vi "Main.vi"() -> ()   [LabVIEW 2018, in "HW Interaction.lvlib"]
doc: "This template is based off of the Queued Message Handler design pattern and the Queued Message Handler project template that ships with LabVIEW.\n\nThe main difference is that the queue is private to this module and communication between modules is performed via Broadcast and Request events.\n\nRequest events are wrapped in public API methods and are handled in the Event Handling Loop (EHL) of this VI. Any module can register for Broadcast events sent by this module. The EHL generates messages based on user interface actions.\n\nThe Message Handling Loop (MHL) processes messages generated by the EHL, or by other messages. The messages are string values, so new messages can be added easily to the Message Cases case structure in the MHL. Each message cluster can also provide an optional value for Message Data, which is a variant that can be converted to whatever message-specific data is required.\n_____\nBased on Delacor QMH Project Template 4.2.1.64."
uses:
  HW Interaction.lvlib
  <vilib>/Delacor/Delacor QMH/Libraries/Module Admin_class/Delacor_lib_QMH_Module Admin.lvclass
  Private API/Data.lvclass
  <vilib>/Delacor/Delacor QMH/Libraries/Message Queue_class/Delacor_lib_QMH_Message Queue.lvclass/Delacor_lib_QMH_Message Queue.ctl
  Stop Argument--cluster.ctl
  <vilib>/Delacor/Delacor QMH/Libraries/Module Admin_class/Delacor_lib_QMH_Module Admin.lvclass/Delacor_lib_QMH_Module Admin.ctl
  Prepare to Exit Argument--cluster.ctl
  HW Init Argument--cluster.ctl
  Public API/Typedefs/CTL_Port_connection_type.ctl
  SubVi's/Controls/CTL_Acquisition_speed_selector.ctl
  <vilib>/Utility/miscctls.llb/LVPointTypeDef.ctl
  Private API/Data.lvclass/Data.ctl
  HW Init Outcome Argument--cluster.ctl
  Public API/Typedefs/CTL_Sensor_board_type_(size).ctl
  Private API/Typedefs/CTL_HW_Interaction_Commands.ctl
  <vilib>/Delacor/Delacor QMH/Libraries/Message Queue_class/Delacor_lib_QMH_Enqueue Message (Single).vi
  <vilib>/Delacor/Delacor QMH/Libraries/Module Admin_class/Delacor_lib_QMH_Get External Launch.vi
  Private API/Methods/Write Status.vi
  Private API/Methods/Write FW Version.vi
  Private API/Methods/Write Sync capability.vi
  Private API/Methods/Write Port Opened.vi
  Private API/Methods/Write Sensor board type.vi
  Private API/Methods/Write HW set FPS.vi
  Private API/Methods/Write Serial Port.vi
  Private API/Methods/Read All Port Info.vi
  <vilib>/Utility/error.llb/Error Cluster From Error Code.vi
  <vilib>/ErrorRing/Error Ring.xnode
  <vilib>/Delacor/Delacor QMH/Libraries/Message Queue_class/Delacor_lib_QMH_Message Queue.lvclass
  Common_Resources.lvlib
panel:
  in  "Simulate MHL Error":bool
  in  "Simulate EHL Error":bool
  out "error out":errorcluster
  in  "Module Admin":refnum<class "Delacor_lib_QMH_Module Admin.lvclass">
  out "Status":string
  # "HW Interaction Module"
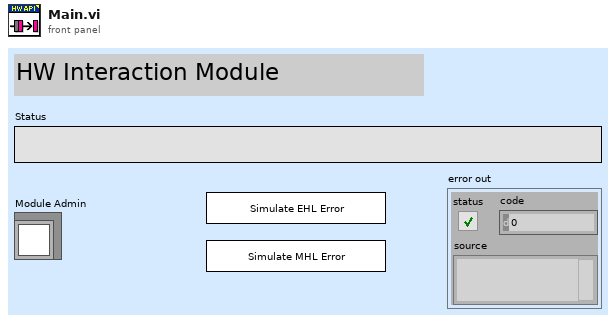
[diagram p1: front panel]
types:
  T1 = typedef "HW Interaction.lvlib/Request Events--cluster.ctl" = cluster{"Stop Module":refnum<user-event>, "Show Panel":refnum<user-event>, "Hide Panel":refnum<user-event>, "Get Module Execution Status":refnum<user-event>, "Show Diagram":refnum<user-event>, "Prepare to Exit":refnum<user-event>, "HW Init":refnum<user-event>}
  T2 = enum32{"invalid lock state", "Not Locked", "Locked (No Password)", "Password-protected"}
  T3 = typedef "HW Interaction.lvlib/Stop Argument--cluster.ctl" = cluster{"Origin":string, "Exit via Stop Module Req?":bool, "Wait for Module to stop?":bool}
  T4 = typedef "HW Interaction.lvlib/Prepare to Exit Argument--cluster.ctl" = cluster{"Origin":string}
  T5 = typedef "HW Interaction.lvlib/HW Init Argument--cluster.ctl" = cluster{"Port Type":T6, "Port Address":string, "Acquisition FPS":T7}
  T6 = typedef "HW Interaction.lvlib/CTL_Port_connection_type.ctl" = enum16{"Serial (VISA)", "TCP/IP"}
  T7 = typedef "Common_Resources.lvlib/CTL_Acquisition_speed_selector.ctl" = enum16{"Max", "Optimal", "Eco"}
  T8 = typedef "LVPointTypeDef.ctl" = cluster{"Horizontal":i16, "Vertical":i16}
  T9 = enum32{"Invalid", "Standard", "Closed", "Hidden", "Minimized", "Maximized"}
  T10 = typedef "HW Interaction.lvlib/HW Init Outcome Argument--cluster.ctl" = cluster{"Outcome":cluster{"HW Init OK?":bool, "Sensor board type":T11, "FW Version":string, "HW set FPS":dbl, "Sync capability":u8}}
  T11 = typedef "HW Interaction.lvlib/CTL_Sensor_board_type_(size).ctl" = enum16{"Small", "Large"}
  T12 = typedef "HW Interaction.lvlib/CTL_HW_Interaction_Commands.ctl" = enum16{"None", "Acquisition Stop", "Connection Stop and Close"}
  T13 = cluster{"HW Init OK?":bool, "Sensor board type":T11, "FW Version":string, "HW set FPS":dbl, "Sync capability":u8}
  T14 = cluster{"Port Type":T6, "VISA resource name out":refnum<visa-resource-name>, string}
  T15 = cluster{"Type":T6, "Serial Port":refnum<visa-resource-name>, "IP Address":string}
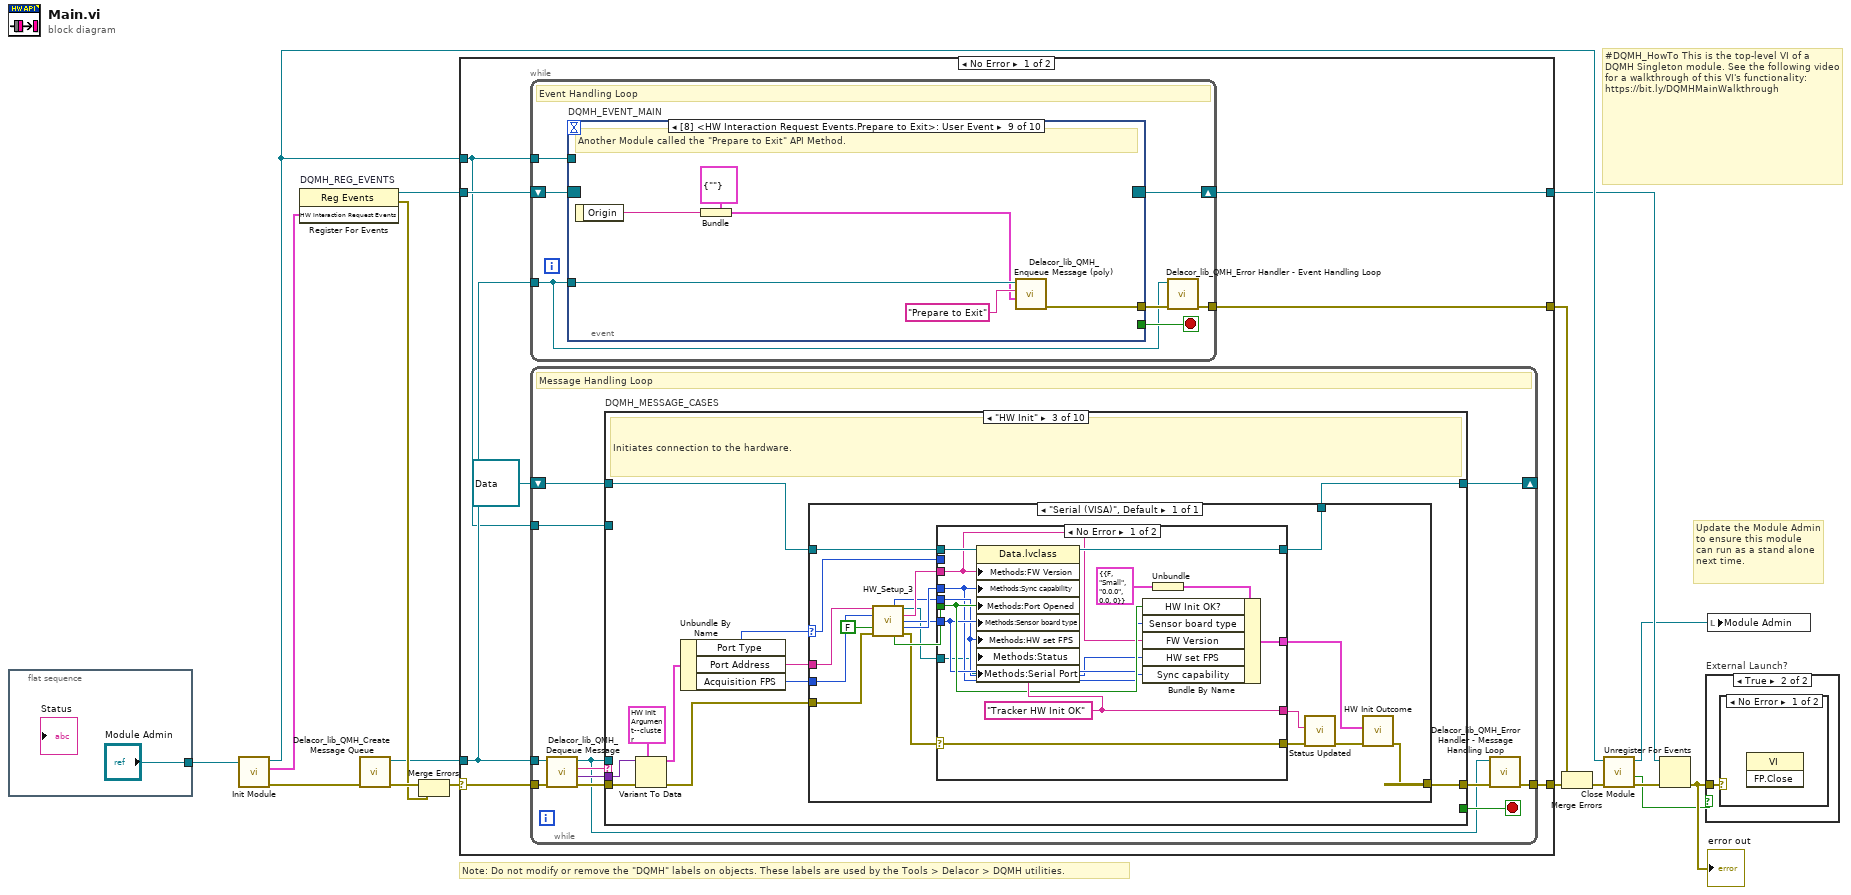
[diagram p0: block diagram]
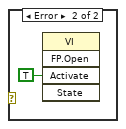
[diagram p3: hidden frame]
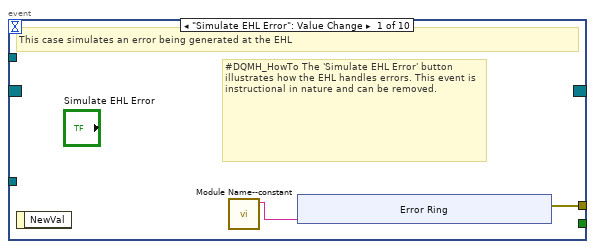
[diagram p4: hidden frame]
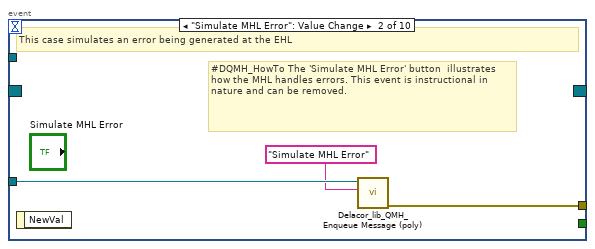
[diagram p5: hidden frame]
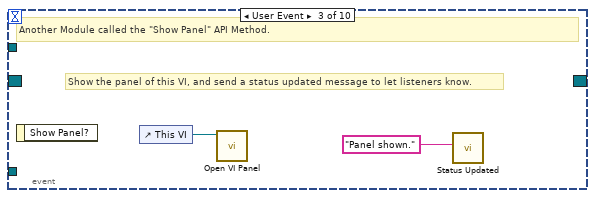
[diagram p6: hidden frame]
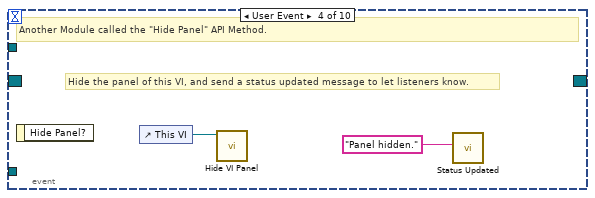
[diagram p7: hidden frame]
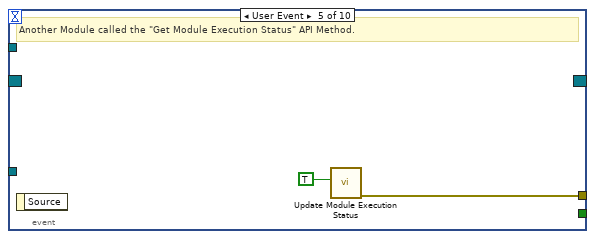
[diagram p8: hidden frame]
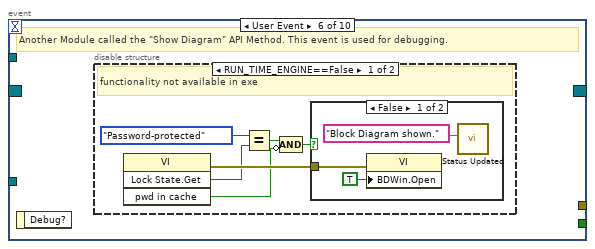
[diagram p9: hidden frame]
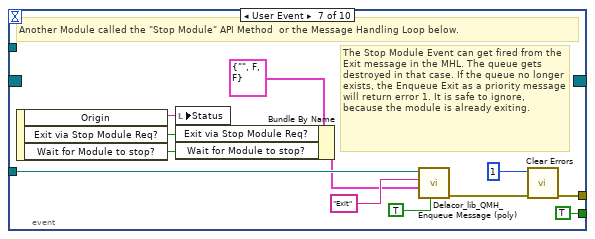
[diagram p12: hidden frame]
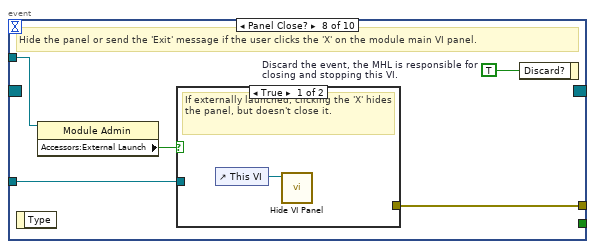
[diagram p13: hidden frame]
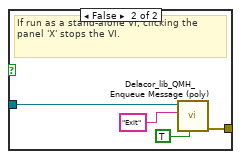
[diagram p14: hidden frame]
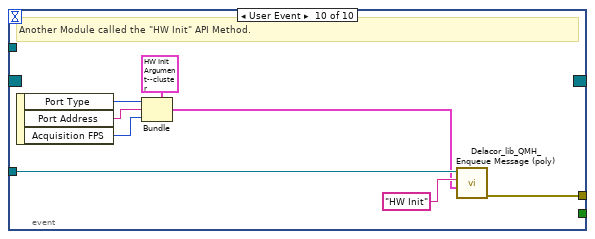
[diagram p15: hidden frame]
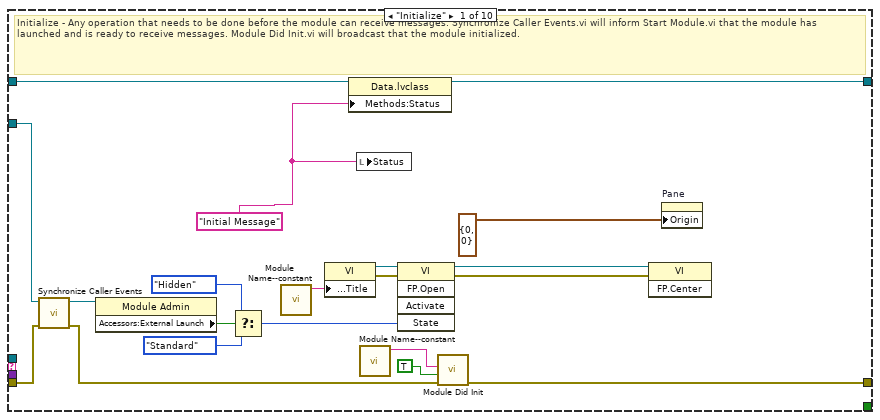
[diagram p16: hidden frame]
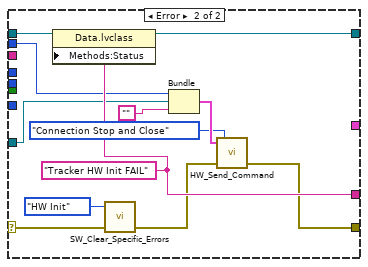
[diagram p18: hidden frame]
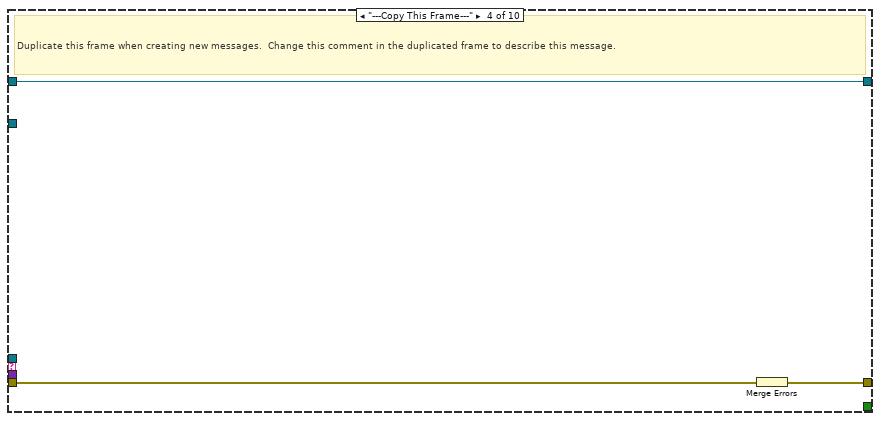
[diagram p19: hidden frame]
diagram:
  # "#DQMH_HowTo This is the top-level VI of a DQMH Singleton module. See the following video for a walkthrough of this VI's functionality: https://bit.ly/DQMHMainWalkthrough"
  # "Note: Do not modify or remove the \"DQMH\" labels on objects. These labels are used by the Tools > Delacor > DQMH utilities."
  # "Update the Module Admin to ensure this module can run as a stand alone next time."
  n1 = flat-sequence {
    tunnel: ["Module Admin"] -> w1
    frame #0 {
    }
  }
  n2 = call "Init Module.vi"("Singleton Module Admin in"=w1) -> ("error out"=w16:errorcluster, "HW Interaction Request Events"=w5:T1, "Singleton Module Admin out"=w8:refnum<class "Delacor_lib_QMH_Module Admin.lvclass">)  [unwired: 8 in]
  n3 = register-events "DQMH_REG_EVENTS"(w5) -> (reference out=w6:refnum<event-registration>, error out=w9:errorcluster)  [unwired: 2 in]
  n4 = call <vilib>:"Delacor_lib_QMH_Create Message Queue.vi"("error in (no error)"=w16) -> ("error out"=w11:errorcluster, "Message Queue"=w4:refnum<class "Delacor_lib_QMH_Message Queue.lvclass">)  [unwired: 9 in]
  n5 = Merge Errors(w11, w9) -> (w10:errorcluster)
  n6 = case shown="No Error" w10 {
    selector: w10 -> [w24 w274]
    tunnel: [w26 w274] -> w17
    tunnel: [w23 w271] -> w7
    tunnel: w6 -> [w22 w271]
    tunnel: w4 -> [w21 _]
    tunnel: [w25 _] -> w14
    tunnel: w8 -> [w20 w267]
    frame No Error {
      n7 = while {
        tunnel: w21 -> [w27]
        shift-right: [w30] -> w23
        shift-left: w22 -> [w31]
        tunnel: [w32] -> w25
        tunnel: w20 -> [w28]
        stop <- w29 stop-if-true
        # "Event Handling Loop"
        n8 = event "DQMH_EVENT_MAIN" shown="[8] <HW Interaction Request Events.Prepare to Exit>: User Event" {
          selector: w31 -> [_ _ _ _ _ _ _ _ _ _]
          dyn-events: [_ _ _ _ _ _ _ _ _ _] -> w30
          timeout: _ -> [_ _ _ _ _ _ _ _ _ _]
          tunnel: [_ _ _ _ _ _ TRUE ("Discard?") _ _ _] -> w29
          tunnel: w27 -> [_ w44 _ _ _ _ w68 w75 w88 w96]
          tunnel: [w35 w45 _ _ w51 _ w71 w77 w83 w89] -> w33
          tunnel: w28 -> [_ _ _ _ _ _ _ w74 _ _]
          event "Simulate EHL Error": Value Change {
            # "#DQMH_HowTo The 'Simulate EHL Error' button  illustrates how the EHL handles errors. This event is instructional in nature and can be removed."
            # "This case simulates an error being generated at the EHL"
            n9 = event-data() -> ()  [unwired: 1 in, 1 out]
            n10 = call "Module Name--constant.vi"() -> ("Module Name"=w34:string)  [unwired: 11 in]
            n11 = xnode "Error Ring"("parameter 0"=w34) -> ("error out"=w35:errorcluster)
          }
          event "Simulate MHL Error": Value Change {
            # "#DQMH_HowTo The 'Simulate MHL Error' button  illustrates how the MHL handles errors. This event is instructional in nature and can be removed."
            # "This case simulates an error being generated at the EHL"
            n12 = event-data() -> ()  [unwired: 1 in, 1 out]
            n13 = call-poly <vilib>:"Delacor_lib_QMH_Enqueue Message (poly).vi"("Message"="Simulate MHL Error", "Message Queue in"=w44) -> ("error out"=w45:errorcluster)  [unwired: 8 in, 1 out]
          }
          event User Event {
            # "Show the panel of this VI, and send a status updated message to let listeners know."
            # "Another Module called the \"Show Panel\" API Method."
            n14 = event-data() -> ()  [unwired: 1 in, 1 out]
            n15 = control-ref of="This VI"() -> (w47:refnum<vi>)
            n16 = call "Open VI Panel.vi"("VI"=w47) -> ()  [unwired: 10 in, 1 out]
            n17 = call "Status Updated.vi"("Status"="Panel shown." ("format string")) -> ()  [unwired: 10 in, 1 out]
          }
          event User Event {
            # "Hide the panel of this VI, and send a status updated message to let listeners know."
            # "Another Module called the \"Hide Panel\" API Method."
            n18 = event-data() -> ()  [unwired: 1 in, 1 out]
            n19 = control-ref of="This VI"() -> (w49:refnum<vi>)
            n20 = call "Hide VI Panel.vi"("VI"=w49) -> ()  [unwired: 10 in, 1 out]
            n21 = call "Status Updated.vi"("Status"="Panel hidden." ("format string")) -> ()  [unwired: 10 in, 1 out]
          }
          event User Event {
            # "Another Module called the \"Get Module Execution Status\" API Method."
            n22 = event-data() -> ()  [unwired: 1 in, 1 out]
            n23 = call "Update Module Execution Status.vi"("Running?"=TRUE) -> ("error out"=w51:errorcluster)  [unwired: 10 in]
          }
          event User Event {
            # "Another Module called the \"Show Diagram\" API Method. This event is used for debugging."
            n24 = event-data() -> ()  [unwired: 1 in, 1 out]
            n25 = disable-structure shown="RUN_TIME_ENGINE==False" {
              frame condition #0 (active) {
                # "functionality not available in exe"
                n26 = invoke class="VI" method="Lock State.Get"() -> (error out=w57:errorcluster, "Get Lock State"=w56:T2, "pwd in cache"=w53:bool)  [unwired: 4 in, 1 out]
                n27 = Equal?(x=T2."Password-protected", y=w56) -> (x = y?=w54:bool)
                n28 = Compound Arithmetic op=AND(w54, invert w53) -> (w52:bool)
                n29 = case shown="False" w52 {
                  tunnel: w57 -> [w60 _]
                  frame False {
                    n30 = property class="VI"(error in=w60, "BDWin.Open"=TRUE ("Block Diagram Window:Open")) -> ()  [unwired: 1 in, 2 out]
                    n31 = call "Status Updated.vi"("Status"="Block Diagram shown." ("format string")) -> ()  [unwired: 10 in, 1 out]
                  }
                  frame True {
                    # "Password-protected VI, and the password is not in the cache. Do not show the diagram."
                  }
                }
              }
              frame condition #1 {
              }
            }
          }
          event User Event {
            # "The Stop Module Event can get fired from the Exit message in the MHL. The queue gets destroyed in that case. If the queue no longer exists, the Enqueue Exit as a priority message will return error 1. It is safe to ignore, because the module is already exiting."
            # "Another Module called the \"Stop Module\" API Method  or the Message Handling Loop below."
            n32 = event-data() -> ("Origin"=w67:string, "Exit via Stop Module Req?"=w63:bool, "Wait for Module to stop?"=w62:bool)  [unwired: 1 in]
            n33 = local write "Status"(w67) -> ()
            n34 = Bundle By Name(cluster=T3 {"Origin"="", "Exit via Stop Module Req?"=FALSE, "Wait for Module to stop?"=FALSE} ("Stop Argument"), "Exit via Stop Module Req?"=w63, "Wait for Module to stop?"=w62) -> (w61:T3)
            n35 = call-poly <vilib>:"Delacor_lib_QMH_Enqueue Message (poly).vi"("Priority Message? (F)"=TRUE, "Message Data"=w61, "Message"="Exit", "Message Queue in"=w68) -> ("error out"=w72:errorcluster)  [unwired: 6 in, 1 out]
            n36 = call <vilib>:"Clear Errors.vi"("error in (no error)"=w72, "specific error code to clear (0: all)"=1) -> ("error out"=w71:errorcluster)  [unwired: 4 in, 1 out]
          }
          event Panel Close? {
            w76 = TRUE  # Discard the event, the MHL is responsible for closing and stopping this VI.
            # "Hide the panel or send the 'Exit' message if the user clicks the 'X' on the module main VI panel."
            n37 = event-data() -> ()  [unwired: 1 in, 1 out]
            n38 = property class="Module Admin"(reference=w74) -> ("Accessors:External Launch"=w73:bool)  [unwired: 1 in, 2 out]
            n39 = case shown="True" w73 {
              tunnel: w75 -> [_ w81]
              tunnel: [_ w82] -> w77
              frame True {
                # "If externally launched, clicking the 'X' hides the panel, but doesn't close it."
                n40 = control-ref of="This VI"() -> (w78:refnum<vi>)
                n41 = call "Hide VI Panel.vi"("VI"=w78) -> ()  [unwired: 10 in, 1 out]
              }
              frame False {
                # "If run as a stand-alone VI, clicking the panel 'X' stops the VI."
                n42 = call-poly <vilib>:"Delacor_lib_QMH_Enqueue Message (poly).vi"("Priority Message? (F)"=TRUE, "Message"="Exit", "Message Queue in"=w81) -> ("error out"=w82:errorcluster)  [unwired: 7 in, 1 out]
              }
            }
            n43 = event-data("Discard?"=w76) -> ()  [unwired: 1 in, 1 out]
          }
          event User Event {
            # "Another Module called the \"Prepare to Exit\" API Method."
            n44 = event-data() -> ("Origin"=w84:string)  [unwired: 1 in]
            n45 = Bundle(cluster=T4 {"Origin"=""} ("Prepare to Exit Argument"), "Origin"=w84) -> (w85:T4)
            n46 = call-poly <vilib>:"Delacor_lib_QMH_Enqueue Message (poly).vi"("Message Data"=w85, "Message"="Prepare to Exit", "Message Queue in"=w88) -> ("error out"=w83:errorcluster)  [unwired: 7 in, 1 out]
          }
          event User Event {
            # "Another Module called the \"HW Init\" API Method."
            n47 = event-data() -> ("Port Type"=w92:T6, "Port Address"=w91:string, "Acquisition FPS"=w90:T7)  [unwired: 1 in]
            n48 = Bundle(cluster=T5 {"Port Type"=enum."Serial (VISA)", "Port Address"="", "Acquisition FPS"=enum."Optimal"} ("HW Init Argument"), "Port Type"=w92, "Port Address"=w91, "Acquisition FPS"=w90) -> (w93:T5)
            n49 = call-poly <vilib>:"Delacor_lib_QMH_Enqueue Message (poly).vi"("Message Data"=w93, "Message"="HW Init", "Message Queue in"=w96) -> ("error out"=w89:errorcluster)  [unwired: 7 in, 1 out]
          }
        }
        n50 = call-dynamic "Delacor_lib_QMH_Error Handler - Event Handling Loop.vi"("error in (no error)"=w33, "Message Queue in"=w27) -> ("dup error in"=w32:errorcluster)  [unwired: 8 in, 1 out]
      }
      n51 = while {
        tunnel: w21 -> [w99]
        shift-right: [w103] -> _
        shift-left: refnum<class "Data.lvclass"> refnum ("HW Interaction.lvlib:Data.lvclass") -> [w104]
        tunnel: w24 -> [w107]
        tunnel: [w105] -> w26
        tunnel: w20 -> [w97]
        stop <- w102 stop-if-true
        # "Message Handling Loop"
        n52 = call-dynamic "Delacor_lib_QMH_Dequeue Message.vi"("error in (no error)"=w107, "Message Queue in"=w99) -> ("error out"=w106:errorcluster, "Message Data"=w100:variant, "Message"=w101:string, "Message Queue out"=w98:refnum<class "Delacor_lib_QMH_Message Queue.lvclass">)  [unwired: 6 in]
        n53 = case "DQMH_MESSAGE_CASES" shown="\"HW Init\"" w101 {
          selector: w101 -> [_ _ _ _ _ _ _ _ _ w254]
          tunnel: w98 -> [_ _ _ _ _ _ w205 _ w246 _]
          tunnel: w106 -> [w126 w130 w141 w188 w190 w195 w212 w237 w252 w256]
          tunnel: [w124 w130 w133 w187 w190 w194 w208 w233 w249 w257] -> w108
          tunnel: w104 -> [w111 w129 w132 w186 w189 w192 w207 w230 w245 w255]
          tunnel: [w109 w129 w131 w186 w189 w192 w207 w230 w245 w255] -> w103
          tunnel: [_ _ _ _ _ _ _ _ w244 _] -> w102
          tunnel: w100 -> [_ _ w140 _ _ _ w206 w236 w243 _]
          tunnel: w97 -> [w116 _ _ _ _ _ w204 _ w238 _]
          frame "Initialize" {
            w110 = "Initial Message" ("Initial Message")
            # "Initialize - Any operation that needs to be done before the module can receive messages. Synchronize Caller Events.vi will inform Start Module.vi that the module has launched and is ready to receive messages. Module Did Init.vi will broadcast that the module initialized."
            n54 = call "Synchronize Caller Events.vi"("error in (no error)"=w126, "Singleton Module Admin in"=w116) -> ("error out"=w125:errorcluster, "Singleton Module Admin out"=w113:refnum<class "Delacor_lib_QMH_Module Admin.lvclass">)  [unwired: 8 in]
            n55 = property class="Module Admin"(reference=w113) -> ("Accessors:External Launch"=w120:bool)  [unwired: 1 in, 2 out]
            n56 = Select(t=T9."Hidden" ("State"), s=w120, f=T9."Standard" ("State")) -> (s? t:f=w117:T9)
            n57 = call "Module Name--constant.vi"() -> ("Module Name"=w123:string)  [unwired: 11 in]
            n58 = property class="VI"("Front Panel.Title"=w123) -> (reference out=w122:refnum<vi>, error out=w128:errorcluster)  [unwired: 2 in]
            n59 = property class="Data.lvclass"(reference=w111, "Methods:Status"=w110) -> (reference out=w109:refnum<class "Data.lvclass">)  [unwired: 1 in, 1 out]
            n60 = local write "Status"(w110) -> ()
            n61 = call "Module Name--constant.vi"() -> ("Module Name"=w114:string)  [unwired: 11 in]
            n62 = invoke class="VI" method="FP.Open"(reference=w122, error in=w128, "State"=w117) -> (reference out=w121:refnum<vi>, error out=w127:errorcluster)  [unwired: 2 in, 3 out]
            n63 = call "Module Did Init.vi"("error in (no error)"=w125, "Initialized?"=TRUE, "Origin"=w114) -> ("error out"=w124:errorcluster)  [unwired: 8 in]
            n64 = invoke class="VI" method="FP.Center"(reference=w121, error in=w127) -> ()  [unwired: 1 in, 3 out]
            n65 = property on="Pane" class="Pane"("Origin"=T8 {"Horizontal"=0, "Vertical"=0}) -> ()  [unwired: 2 in, 2 out]
          }
          frame "--- Module Specific ---" {
            # "Separator -- The following cases handle messages specific to this Module."
          }
          frame "HW Init" {
            # "Initiates connection to the hardware."
            n66 = Variant To Data(error in=w141, type=T5 {"Port Type"=enum."Serial (VISA)", "Port Address"="", "Acquisition FPS"=enum."Optimal"} ("HW Init Argument"), Variant=w140) -> (data=w138:T5, error out=w134:errorcluster)
            n67 = Unbundle By Name(w138) -> ("Port Type"=w137:T6, "Port Address"=w136:string, "Acquisition FPS"=w135:T7)
            n68 = case shown="\"Serial (VISA)\", Default" w137 {
              selector: w137 -> [w142]
              tunnel: w136 -> [w160]
              tunnel: w135 -> [w159]
              tunnel: w134 -> [w158]
              tunnel: [w146] -> w133
              tunnel: w132 -> [w157]
              tunnel: [w149] -> w131
              frame "Serial (VISA)", Default {
                n69 = call "HW_Setup_3.vi"("VISA resource name in"=w160, "Acquisition FPS"=w159, "Close port? (F)"=FALSE, "error in"=w158) -> ("FPS status"=w152:i32, "VISA resource name out"=w143:refnum<visa-resource-name>, "HW information"=w156:string, "SB type (size)"=w153:T11, "Sync capability"=w155:u8, "Instrument OK?"=w154:bool, "error out"=w151:errorcluster)  [unwired: 5 in]
                n70 = case shown="No Error" w151 {
                  selector: w151 -> [w172 w185]
                  tunnel: w157 -> [w173 w183]
                  tunnel: w156 -> [w163 _]
                  tunnel: w155 -> [w162 _]
                  tunnel: w154 -> [w166 _]
                  tunnel: w153 -> [w165 _]
                  tunnel: w152 -> [w164 _]
                  tunnel: [w172 w179] -> w150
                  tunnel: [w171 w182] -> w149
                  tunnel: [w170 w181] -> w148
                  tunnel: [w168 _] -> w145
                  tunnel: w143 -> [w161 w177]
                  tunnel: w142 -> [_ w178]
                  frame No Error {
                    w170 = "Tracker HW Init OK"
                    n71 = property class="Data.lvclass"(reference=w173, "Methods:FW Version"=w163, "Methods:Sync capability"=w162, "Methods:Port Opened"=w166, "Methods:Sensor board type"=w165, "Methods:HW set FPS"=w164, "Methods:Status"=w170, "Methods:Serial Port"=w161) -> (reference out=w171:refnum<class "Data.lvclass">)  [unwired: 1 in, 1 out]
                    n72 = Unbundle(T10 {"Outcome"={"HW Init OK?"=FALSE, "Sensor board type"=enum."Small", "FW Version"="0.0.0", "HW set FPS"=0.0, "Sync capability"=0}} ("HW Init Outcome Argument")) -> ("Outcome"=w167:T13)
                    n73 = Bundle By Name(cluster=w167, "HW Init OK?"=w166, "Sensor board type"=w165, "FW Version"=w163, "HW set FPS"=w164, "Sync capability"=w162) -> (w168:T13)
                  }
                  frame Error {
                    w181 = "Tracker HW Init FAIL"
                    n74 = property class="Data.lvclass"(reference=w183, "Methods:Status"=w181) -> (reference out=w182:refnum<class "Data.lvclass">)  [unwired: 1 in, 1 out]
                    n75 = call "SW_Clear_Specific_Errors.vi"("Error In"=w185, "Code section"=enum16{"Not Specified", "HW Init"}."HW Init") -> ("Error Out"=w180:errorcluster)  [unwired: 2 in, 1 out]
                    n76 = Bundle("Port Type"=w178, "VISA resource name out"=w177, "") -> (w175:T14)  [unwired: 1 in]
                    n77 = call "HW_Send_Command.vi"("Error In"=w180, "HW Command"=CTL_HW_Interaction_Commands."Connection Stop and Close", "Port info in"=w175) -> ("Error Out"=w179:errorcluster)  [unwired: 2 out]
                  }
                }
                n78 = call "Status Updated.vi"("error in (no error)"=w150, "Status"=w148) -> ("error out"=w147:errorcluster)  [unwired: 9 in]
                n79 = call "HW Init Outcome.vi"("error in (no error)"=w147, "Outcome"=w145) -> ("error out"=w146:errorcluster)  [unwired: 9 in]
              }
            }
          }
          frame "---Copy This Frame---" {
            # "Duplicate this frame when creating new messages.  Change this comment in the duplicated frame to describe this message."
            n80 = Merge Errors(w188) -> (w187:errorcluster)
          }
          frame "--- Exit and Error Handling---" {
            # "Separator - The following cases handle errors and exit messages."
          }
          frame "Simulate MHL Error" {
            # "#DQMH_HowTo The 'Simulate MHL Error' button  illustrates how the MHL handles errors. This event is instructional in nature and can be removed."
            # "Simulate an error occurring at the MHL"
            n81 = call "Module Name--constant.vi"() -> ("Module Name"=w191:string)  [unwired: 11 in]
            n82 = xnode "Error Ring"("parameter 0"=w191) -> ("error out"=w193:errorcluster)
            n83 = Merge Errors(w195, w193) -> (w194:errorcluster)
          }
          frame "Error" {
            # "#CodeRecommended - If you ever change the name of this \"Error\" message, you'll need to update the name in the Check Loop Error.vi as well."
            # "#CodeRecommended - If the module is running in standalone mode (External Launch = FALSE), this code will pop up an error dialog and call the 'Exit' message if an error occurs. Add more fine-grained error handling here."
            # "Error - Check the error message data and respond accordingly. This message is sent by the \"Error Handler\" VIs at the end of each loop in this application."
            n84 = property class="Module Admin"(reference=w204) -> ("Accessors:External Launch"=w203:bool)  [unwired: 1 in, 2 out]
            n85 = Variant To Data(error in=w212, type=errorcluster {"status"=FALSE, "code"=0, "source"=""} ("error constant"), Variant=w206) -> (data=w213:errorcluster, error out=w210:errorcluster)
            n86 = call "Error Reported.vi"("Error"=w213) -> ()  [unwired: 10 in, 1 out]
            n87 = case shown="False" w203 {
              tunnel: [w218 _] -> w209
              tunnel: w205 -> [w216 _]
              tunnel: w213 -> [w217 _]
              frame False {
                n88 = call <vilib>:"Simple Error Handler.vi"("error in (no error)"=w217) -> ()  [unwired: 4 in, 5 out]
                n89 = call-poly <vilib>:"Delacor_lib_QMH_Enqueue Message (poly).vi"("Priority Message? (F)"=TRUE, "Message"="Prepare to Exit", "Message Queue in"=w216) -> ("error out"=w218:errorcluster)  [unwired: 7 in, 1 out]
              }
              frame True {
              }
            }
            n90 = Merge Errors(w210, w209) -> (w208:errorcluster)
            n91 = local write "error out"(w208) -> ()
          }
          frame "Prepare to Exit" {
            # "Initiates exit sequence for HW Interaction module."
            n92 = Variant To Data(error in=w237, type=T4 {"Origin"=""} ("Prepare to Exit Argument"), Variant=w236) -> (data=w234:T4, error out=w231:errorcluster)
            n93 = property class="Data.lvclass"(reference=w230) -> ("Methods:All Port Info"=w229:T15)  [unwired: 1 in, 2 out]
            n94 = call "HW_Send_Command.vi"("Error In"=w231, "HW Command"=CTL_HW_Interaction_Commands."Acquisition Stop", "Port info in"=w229) -> ("Error Out"=w227:errorcluster, "Message"=w226:string, "Port info out"=w224:T15)
            n95 = call "Status Updated.vi"("error in (no error)"=w227, "Status"=w226) -> ("error out"=w225:errorcluster)  [unwired: 9 in]
            n96 = call "HW_Send_Command.vi"("Error In"=w225, "HW Command"=CTL_HW_Interaction_Commands."Connection Stop and Close", "Port info in"=w224) -> ("Error Out"=w221:errorcluster, "Message"=w219:string)  [unwired: 1 out]
            n97 = call "Status Updated.vi"("error in (no error)"=w221, "Status"=w219) -> ("error out"=w220:errorcluster)  [unwired: 9 in]
            n98 = Unbundle By Name(w234) -> ("Origin"=w232:string)
            n99 = call "Stop Module.vi"("Timeout to Wait for Stop (s) (-1: no timeout)"=5.0, "error in (no error)"=w220, "Origin"=w232) -> ("error out"=w233:errorcluster)  [unwired: 8 in]
          }
          frame "Exit" {
            w242 = 91  # 91: not all Exit messages will have an argument
            w244 = TRUE  # Stop the VI
            # "Release the message queue reference"
            # "#CodeNeeded - Add any required cleanup code here"
            # "Exit - Exit the application."
            n100 = Variant To Data(error in=w252, type=T3 {"Origin"="", "Exit via Stop Module Req?"=FALSE, "Wait for Module to stop?"=FALSE} ("Stop Argument"), Variant=w243) -> (data=w240:T3, error out=w248:errorcluster)
            n101 = call <vilib>:"Clear Errors.vi"("error in (no error)"=w248, "specific error code to clear (0: all)"=w242) -> ("error out"=w251:errorcluster)  [unwired: 4 in, 1 out]
            n102 = control-ref of="This VI"() -> (w239:refnum<vi>)
            n103 = call-dynamic "Delacor_lib_QMH_Release Message Queue.vi"("error in (no error)"=w251, "Message Queue"=w246) -> ("error out"=w250:errorcluster)  [unwired: 9 in]
            n104 = call "Handle Exit.vi"("Stop Argument"=w240, "Admin in"=w238, "VI reference"=w239) -> ("error out"=w247:errorcluster)  [unwired: 7 in, 1 out]
            n105 = Merge Errors(w250, w247) -> (w249:errorcluster)
          }
          frame Default {
            # "'Default' case only runs if there is a message that isn't defined in any of the other cases.  Output a programming error."
            n106 = call "Module Name--constant.vi"() -> ("Module Name"=w253:string)  [unwired: 11 in]
            n107 = xnode "Error Ring"("parameter 0"=w254, "parameter 1"=w253) -> ("error out"=w258:errorcluster)
            n108 = Merge Errors(w256, w258) -> (w257:errorcluster)
          }
        }
        n109 = call-dynamic "Delacor_lib_QMH_Error Handler - Message Handling Loop.vi"("error in (no error)"=w108, "Message Queue in"=w98) -> ("dup error in"=w105:errorcluster)  [unwired: 8 in, 1 out]
      }
    }
    frame Error {
      # "Synchronize Caller Events.vi will inform Start Module.vi that the module has launched and will let the code calling Start Module.vi register for broadcasts and would permit the caller receive the broadcast that an error occurred at launch time."
      n110 = call "Synchronize Caller Events.vi"("Singleton Module Admin in"=w267) -> ("error out"=w272:errorcluster)  [unwired: 9 in, 1 out]
      n111 = call "Module Name--constant.vi"() -> ("Module Name"=w270:string)  [unwired: 11 in]
      n112 = Format Into String(format string="An error occurred during initialization. %s is no longer running.", w270) -> (resulting string=w268:string)  [unwired: 2 in, 1 out]
      n113 = Merge Errors(w274, w272) -> (w273:errorcluster)
      n114 = call "Error Reported.vi"("Additional Information"=w268, "Error"=w273) -> ()  [unwired: 9 in, 1 out]
    }
  }
  n115 = Merge Errors(w14, w17) -> (w13:errorcluster)
  n116 = call "Close Module.vi"("error in (no error)"=w13, "Module Admin in"=w8) -> ("error out"=w15:errorcluster, "External Launch"=w2:bool, "Module Admin out"=w3:refnum<class "Delacor_lib_QMH_Module Admin.lvclass">)  [unwired: 7 in]
  n117 = Unregister For Events(event registration refnum=w7, error in=w15) -> (error out=w12:errorcluster)
  "error out" <- w12
  n118 = case "External Launch?" shown="True" w2 {
    tunnel: w12 -> [_ w275]
    frame False {
    }
    frame True {
      n119 = case shown="No Error" w275 {
        frame No Error {
          n120 = invoke class="VI" method="FP.Close"() -> ()  [unwired: 3 in, 3 out]
        }
        frame Error {
          n121 = invoke class="VI" method="FP.Open"("Activate"=TRUE ("Activate?")) -> ()  [unwired: 4 in, 5 out]
        }
      }
    }
  }
  n122 = local write "Module Admin"(w3) -> ()
